vi "parseTemporaryAddressError.vi"(8 "error in (no error)":errorcluster, 10 "ModbusBuffer in":refnum<class "ModbusBuffer.lvclass">, 11 "ILC in":refnum<class "ILC.lvclass">) -> (0 "error out":errorcluster, 2 "ModbusBuffer out":refnum<class "ModbusBuffer.lvclass">, 3 "ILC out":refnum<class "ILC.lvclass">)   [LabVIEW 2016, in "RTILC.lvlib" / "ILC.lvclass"]
uses:
  ILC.lvclass
  Common_RT_Modbus/ModbusBuffer/ModbusBuffer.lvclass
  Common_RT_Modbus/ModbusBuffer/ModbusBuffer.lvclass/ModbusBuffer.ctl
  Common_RT_Modbus/DataTypes/ExceptionCodes.ctl
  ILC.lvclass/ILC.ctl
  Common_RT_Modbus/ModbusBuffer/readTimestampByte.vi
  Common_RT_Modbus/ModbusBuffer/readInstructionByte.vi
  Common_RT_Modbus/RTModbus.lvlib
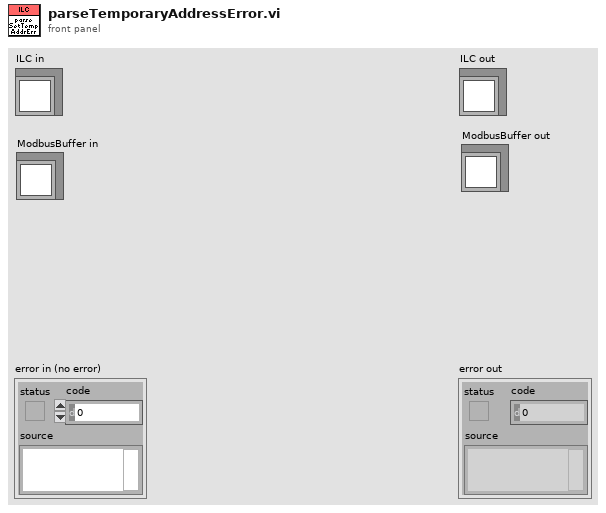
[diagram p1: front panel]
types:
  T1 = typedef "RTModbus.lvlib/ExceptionCodes.ctl" = u16
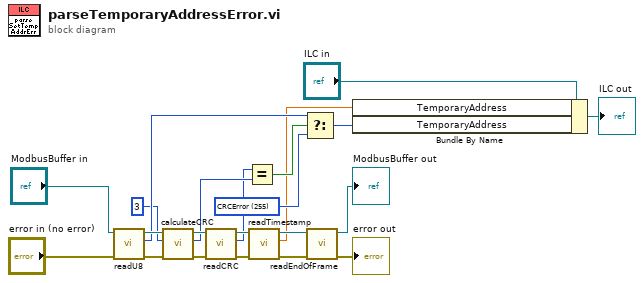
[diagram p0: block diagram]
diagram:
  w19 = T1 255 items=["OK"=0, "IllegalFunction"=1, "IllegalDataAddress"=2, "IllegalDataValue"=3, "SlaveDeviceFailure"=4, "Acknowledge"=5, "SlaveDeviceBusy"=6, "NegativeAcknowledge"=7, "MemoryParityError"=8, "GatewayPathUnavailable"=9, "GatewayTargetDeviceFailedToRespond"=10, "WaitingForResponse"=254, "CRCError"=255] ("f")
  n1 = call "readU8.vi"("error in (no error)"="error in (no error)", "ModbusBuffer in"="ModbusBuffer in") -> ("error out"=w11:errorcluster, "Output"=w10:u8, "ModbusBuffer out"=w12:refnum<class "ModbusBuffer.lvclass">)  [unwired: 7 in]
  n2 = call "calculateCRC.vi"("error in (no error)"=w11, "Length"=3, "ModbusBuffer in"=w12) -> ("error out"=w13:errorcluster, "CRC"=w8:u16, "ModbusBuffer out"=w18:refnum<class "ModbusBuffer.lvclass">)  [unwired: 6 in]
  n3 = call "readCRC.vi"("error in (no error)"=w13, "ModbusBuffer in"=w18) -> ("error out"=w14:errorcluster, "Output"=w7:u16, "ModbusBuffer out"=w17:refnum<class "ModbusBuffer.lvclass">)  [unwired: 7 in]
  n4 = Equal?(x=w7, y=w8) -> (x = y?=w20:bool)
  n5 = call "readTimestamp.vi"("error in (no error)"=w14, "ModbusBuffer in"=w17) -> ("error out"=w15:errorcluster, "Output"=w5:dbl, "ModbusBuffer out"=w16:refnum<class "ModbusBuffer.lvclass">)  [unwired: 7 in]
  n6 = Select(t=w10, s=w20, f=w19) -> (s? t:f=w6:T1)
  n7 = call "readEndOfFrame.vi"("error in (no error)"=w15, "ModbusBuffer in"=w16) -> ("error out"=→"error out":errorcluster, "ModbusBuffer out"=→"ModbusBuffer out":refnum<class "ModbusBuffer.lvclass">)  [unwired: 8 in]
  n8 = Bundle By Name(cluster="ILC in", "TemporaryAddress"=w5, "TemporaryAddress"=w6) -> (→"ILC out":refnum<class "ILC.lvclass">)
